vi "报警值发送回执.vi"(8 "错误 i":errorcluster caption="错误常量", 11 "限值":dbl format="%#_13g") -> (0 "错误 o":errorcluster caption="错误常量", 3 "指令输出":string)   [LabVIEW 2017]
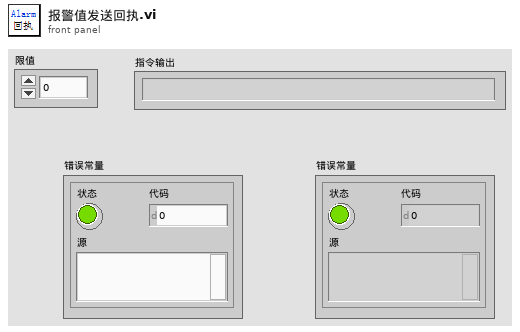
[diagram p1: front panel]
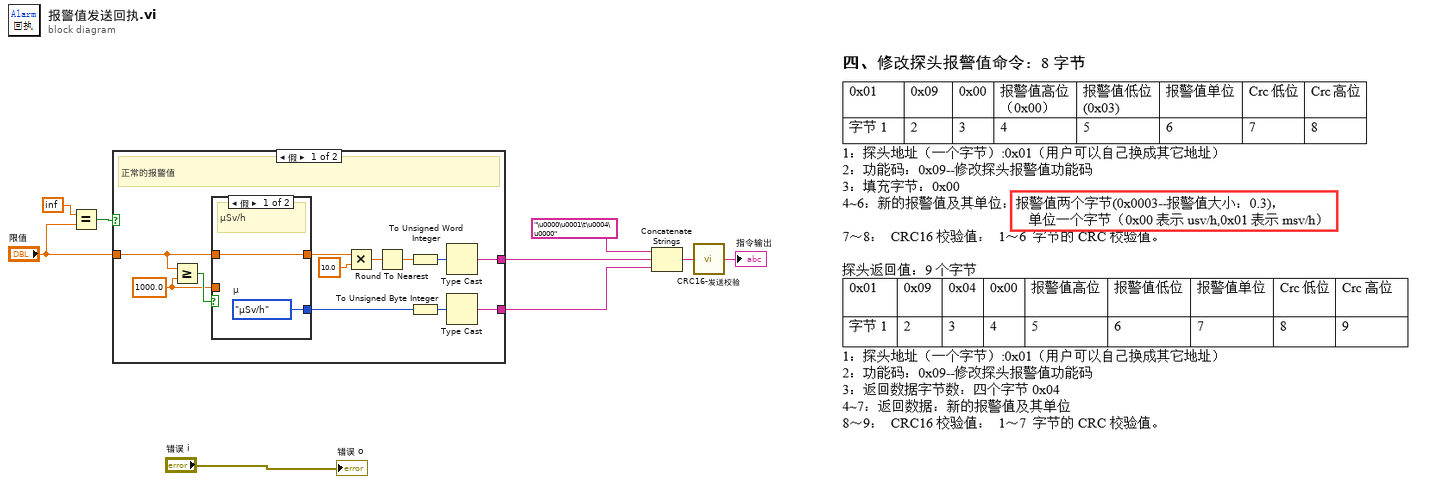
[diagram p0: block diagram]
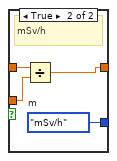
[diagram p2: hidden frame]
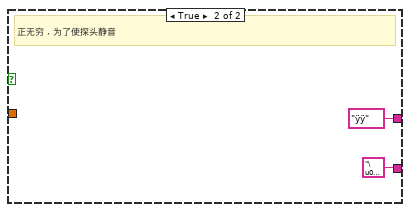
[diagram p3: hidden frame]
diagram:
  n1 = Equal?(x=inf, y="限值") -> (x = y?=w9:bool)
  n2 = case shown="假" w9 {
    tunnel: [w12 "\u0001"] -> w4
    tunnel: [w11 "ÿÿ"] -> w6
    tunnel: "限值" -> [w10 _]
    frame False {
      w20 = 1000.0 ("y")
      # "正常的报警值"
      n3 = Greater Or Equal?(x=w10, y=w20) -> (x >= y?=w21:bool)
      n4 = case shown="假" w21 {
        tunnel: w10 -> [w22 w26]
        tunnel: [w23 w27] -> w14
        tunnel: w20 -> [_ w25]
        tunnel: [w22 w24] -> w19
        frame False {
          w23 = enum8{"μSv/h", "mSv/h"}."μSv/h"  # μ
          # "μSv/h"
        }
        frame True {
          w27 = enum8{"μSv/h", "mSv/h"}."mSv/h"  # m
          # "mSv/h"
          n5 = Divide(x=w26, y=w25) -> (x/y=w24:dbl)
        }
      }
      n6 = Multiply(x=w19, y=10.0) -> (x*y=w16:dbl)
      n7 = Round To Nearest(number=w16) -> (nearest integer value=w15:dbl)
      n8 = To Unsigned Word Integer(number=w15) -> (unsigned 16bit integer=w17:u16)
      n9 = To Unsigned Byte Integer(number=w14) -> (unsigned 8bit integer=w13:u8)
      n10 = Type Cast(x=w17) -> (*(type *) &x=w11:string)  [unwired: 1 in]
      n11 = Type Cast(x=w13) -> (*(type *) &x=w12:string)  [unwired: 1 in]
    }
    frame True {
      # "正无穷 , 为了使探头静音"
    }
  }
  n12 = Concatenate Strings("\u0000\u0001\t\u0004\u0000", w6, w4) -> (w3:string)
  n13 = call "CRC16-发送校验.vi"("净数据"=w3) -> ("完整输出"=→"指令输出":string)
  "错误 o" <- "错误 i"
